vi "Alicat Simplified Driver Example_Multiple Devices with Setpoint.vi"() -> ()   [LabVIEW 2015]
doc: "Simplified example program for initializing the COM port, determining the data frame of up to 26 Alicats, acquiring the data of the same number of Alicats, displaying the data of the one with the selected unit ID, and writing a setpoint to the same selected unit ID.\n\nThis is a slightly more feature rich version of the Alicat Simplified Driver Example, and contains an example of a method for interfacing with up to 26 Alicats on a single COM port by means of for loops with shift registers to handle sequential commands to each included Alicat. This also contains a method to write a setpoint to the same selected unit.\n\nIf coding for multiple Alicats on a single COM port without the use of for loops with shift registers, ensure that each Alicat command is executed sequentially. Alicat's RS-232/485 does not work if multiple devices are responding simultaneously."
panel:
  in  "Setpoint (for \ndevice selected)":dbl format="%_4g"
  out "Meas. Data (for active device)":T1
  in  "Active Device":u16(ring) items=["A", "B", "C"]
  in  "Device ID's \nto Include:":T2={"A"=TRUE, "B"=FALSE, "C"=FALSE, "D"=FALSE, "E"=FALSE, "F"=FALSE, "G"=FALSE, "H"=FALSE, "I"=FALSE, "J"=FALSE, "K"=FALSE, "L"=FALSE, "M"=FALSE, "N"=FALSE, "O"=FALSE, "P"=FALSE, "Q"=FALSE, "R"=FALSE, "S"=FALSE, "T"=FALSE, "U"=FALSE, "V"=FALSE, "W"=FALSE, "X"=FALSE, "Y"=FALSE, "Z"=FALSE}
  in  "Minimum time between \nreadings [ms] (all units)":u32
  out "Elapsed Time [ms]\n(all units)":dbl caption="Elapsed Time (s)"
  in  "End Program":bool
  out "Error Text":string
  out "Error Present":bool
  out "Range Exceeded":bool
  in  "COM Port Settings":T3={"Baud Rate"=enum."19200", "VISA Sesssion In"="COM1"}
  # "Totalizer Timer"
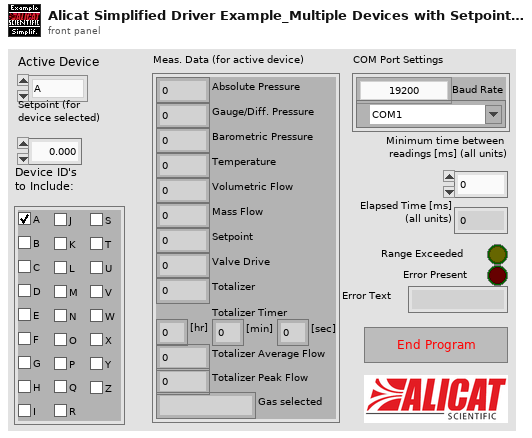
[diagram p1: front panel]
types:
  T1 = cluster{"Absolute Pressure":dbl, "Gauge/Diff. Pressure":dbl, "Barometric Pressure":dbl, "Temperature":dbl, "Volumetric Flow":dbl, "Mass Flow":dbl, "Setpoint":dbl, "Valve Drive":dbl, "Totalizer":dbl, "[hr]":dbl, "[min]":dbl, "[sec]":dbl, "Totalizer Average Flow":dbl, "Totalizer Peak Flow":dbl, "Gas selected":string}
  T2 = cluster{"A":bool, "B":bool, "C":bool, "D":bool, "E":bool, "F":bool, "G":bool, "H":bool, "I":bool, "J":bool, "K":bool, "L":bool, "M":bool, "N":bool, "O":bool, "P":bool, "Q":bool, "R":bool, "S":bool, "T":bool, "U":bool, "V":bool, "W":bool, "X":bool, "Y":bool, "Z":bool}
  T3 = cluster{"Baud Rate":enum8{"2400", "9600", "19200", "38400", "57600", "115200", "Unknown"}, "VISA Sesssion In":refnum<visa-resource-name>}
  T4 = cluster{"Unit ID":string, "Baud Rate":enum8{"2400", "9600", "19200", "38400", "57600", "115200", "Unknown"}, "VISA Sesssion In":refnum<visa-resource-name>}
  T5 = enum8{"2400", "9600", "19200", "38400", "57600", "115200", "Unknown"}
  T6 = cluster{"Absolute Pressure":bool, "Gauge/Diff. Pressure":bool, "Barometric Pressure":bool, "Temperature":bool, "Volumetric":bool, "Mass":bool, "Setpoint":bool, "Valve Drive":bool, "Totalizer":bool, "Totalizer Timer":bool, "Totalizer Average Flow":bool, "Totalizer Peak Flow":bool, "Gas Selected":bool, "Tot. Timer Format":u16}
  T7 = cluster{"Controller Full Scale":dbl, "Controller Select":u16, "Control Range":enum16{"Normal", "Inverted", "Bidirectional", "Unknown"}}
  T8 = cluster{"Controller Full Scale":dbl, "Controller Select":u16, "Control Range":enum16{"Normal", "Inverted", "Bidirectional", "Unknown"}}[]
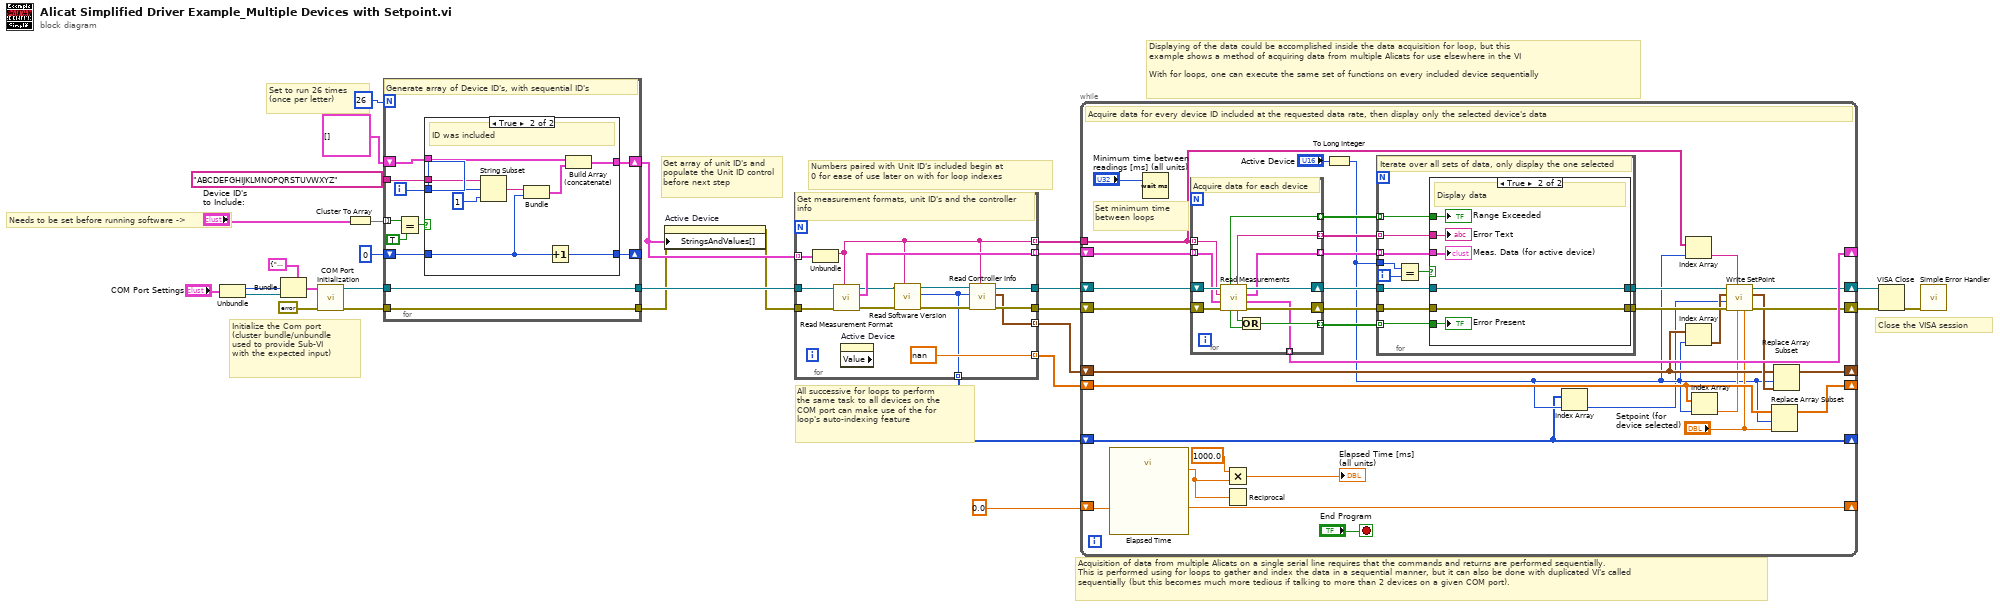
[diagram p0: block diagram]
diagram:
  # "All successive for loops to perform\nthe same task to all devices on the\nCOM port can make use of the for\nloop's auto-indexing feature"
  # "Set to run 26 times\n(once per letter)"
  # "Acquisition of data from multiple Alicats on a single serial line requires that the commands and returns are performed sequentially.\nThis is performed using for loops to gather and index the data in a sequential manner, but it can also be done with duplicated VI's called\nsequentially (but this becomes much more tedious if talking to more than 2 devices on a given COM port)."
  # "Numbers paired with Unit ID's included begin at\n0 for ease of use later on with for loop indexes"
  # "Displaying of the data could be accomplished inside the data acquisition for loop, but this\nexample shows a method of acquiring data from multiple Alicats for use elsewhere in the VI\n\nWith for loops, one can execute the same set of functions on every included device sequentially"
  # "Get array of unit ID's and populate the Unit ID control before next step"
  # "Needs to be set before running software ->"
  # "Close the VISA session"
  # "Initialize the Com port\n(cluster bundle/unbundle\nused to provide Sub-VI \nwith the expected input)"
  n1 = Unbundle("COM Port Settings") -> ("Baud Rate"=w22:T5, "VISA Sesssion In"=w21:refnum<visa-resource-name>)
  n2 = Bundle(cluster=T4 {"Unit ID"="A", "Baud Rate"=enum."19200", "VISA Sesssion In"="COM1"} ("Communication Settings"), "Baud Rate"=w22, "VISA Sesssion In"=w21) -> (w20:T4)  [unwired: 1 in]
  n3 = call "COM Port Initialization.vi"("error in (no error)"=errorcluster {"status"=FALSE, "code"=0, "source"=""}, "Communication Settings"=w20) -> ("error out"=w13:errorcluster, "VISA Session Out"=w12:refnum<visa-resource-name>)  [unwired: 8 in]
  n4 = Cluster To Array(cluster="Device ID's \nto Include:") -> (array=w16:bool[])
  n5 = for {
    N: 26 -> [_]
    tunnel: "ABCDEFGHIJKLMNOPQRSTUVWXYZ" -> [w40]
    tunnel: w16 -> [w33] mode=indexing
    shift-right: [w32] -> _
    shift-left: u16 0 ("length (rest)") -> [w38]
    shift-right: [w37] -> w10
    shift-left: cluster{string, u16}[] [] -> [w36]
    tunnel: w13 -> [w31]
    tunnel: w12 -> [w30]
    tunnel: [w31] -> w3
    tunnel: [w30] -> w11
    i -> [w39]
    # "Generate array of Device ID's, with sequential ID's"
    n6 = Equal?(x=w33, y=TRUE) -> (x = y?=w35:bool)
    n7 = case shown="True" w35 {
      tunnel: w40 -> [_ w51]
      tunnel: w39 -> [_ w50]
      tunnel: w38 -> [w41 w43]
      tunnel: [w42 w46] -> w37
      tunnel: w36 -> [w42 w44]
      tunnel: [w41 w47] -> w32
      frame False {
        # "ID was not included"
      }
      frame True {
        # "ID was included"
        n8 = String Subset(string=w51, offset (0)=w50, length (rest)=1 ("length (rest)")) -> (substring=w48:string)
        n9 = Bundle(w48, "length (rest)"=w43) -> (w45:cluster{string, "length (rest)":u16})  [unwired: 1 in]
        n10 = Increment(x=w43) -> (x+1=w47:u16)
        n11 = Build Array (concatenate)(w44, w45) -> (w46:cluster{string, "length (rest)":u16}[])
      }
    }
  }
  n12 = property on="Active Device" class="Ring (strict)"(error in=w3, "StringsAndValues[]"=w10) -> (error out=w2:errorcluster)  [unwired: 1 in, 1 out]
  n13 = for {
    tunnel: w11 -> [w64]
    tunnel: [w61] -> w7
    tunnel: w2 -> [w65]
    tunnel: [w60] -> w6
    tunnel: w10 -> [w62] mode=indexing
    tunnel: [w63] -> w9 mode=indexing
    tunnel: [w53] -> w8 mode=indexing
    tunnel: [w59] -> w5 mode=indexing
    tunnel: [nan ("Setpoint")] -> w4 mode=indexing
    tunnel: [w52] -> w1 mode=indexing
    # "Get measurement formats, unit ID's and the controller info"
    n14 = Unbundle(w62) -> (w53:string)  [unwired: 1 out]
    n15 = call "Read Measurement Format.vi"("Unit ID (A)"=w53, "error in"=w65, "VISA Session In"=w64) -> ("error out"=w56:errorcluster, "Data Frame Format"=w63:T6, "VISA Session Out"=w57:refnum<visa-resource-name>)  [unwired: 6 in]
    n16 = property on="Active Device" class="Ring (strict)" props=["Value"]() -> ()  [unwired: 2 in, 3 out]
    n17 = call "Read Software Version.vi"("Unit ID (A)"=w53, "error in"=w56, "VISA Session In"=w57) -> ("error out"=w55:errorcluster, "Software Version"=w52:u8, "VISA Session Out"=w54:refnum<visa-resource-name>)  [unwired: 6 in]
    n18 = call "Read Controller Info.vi"("Unit ID (A)"=w53, "error in"=w55, "Software Version"=w52, "VISA Session In"=w54) -> ("error out"=w60:errorcluster, "Controller Info out"=w59:T7, "VISA Session Out"=w61:refnum<visa-resource-name>)  [unwired: 4 in, 1 out]
  }
  n19 = while {
    shift-right: [w97] -> _
    shift-left: 0.0 ("Set Start Time (s)") -> [w100]
    shift-right: [w79] -> w25
    shift-left: w6 -> [w99]
    shift-right: [w80] -> w26
    shift-left: w7 -> [w98]
    tunnel: w8 -> [w71]
    shift-right: [w83] -> _
    shift-left: w9 -> [w91]
    shift-right: [w78] -> _
    shift-left: w5 -> [w76]
    shift-right: [w74] -> _
    shift-left: w4 -> [w73]
    shift-right: [w66] -> _
    shift-left: w1 -> [w66]
    stop <- "End Program" stop-if-true
    # "Set minimum time\nbetween loops"
    # "Acquire data for every device ID included at the requested data rate, then display only the selected device's data"
    n20 = call "Elapsed Time"("Set Start Time (s)"=w100) -> ("Get Start Time (s)"=w97:dbl, "Elapsed Time (s)"=w93:dbl)  [unwired: 11 in, 6 out]
    n21 = Wait (ms)(milliseconds to wait="Minimum time between \nreadings [ms] (all units)") -> ()  [unwired: 1 out]
    n22 = for {
      shift-right: [w129] -> w90
      shift-left: w99 -> [w132]
      shift-right: [w130] -> w89
      shift-left: w98 -> [w131]
      tunnel: w91 -> [w126] mode=indexing
      tunnel: w71 -> [w125] mode=indexing
      tunnel: [w124] -> w88 mode=indexing
      tunnel: [w123] -> w86 mode=indexing
      tunnel: [w122] -> w85 mode=indexing
      tunnel: [w121] -> w84 mode=indexing
      tunnel: [w120] -> w83 mode=indexing
      # "Acquire data for each device"
      n23 = call "Read Measurements.vi"("error in"=w132, "Data Frame Format In"=w126, "Unit ID (A)"=w125, "VISA Session In"=w131) -> ("error out"=w129:errorcluster, "Data Frame Format Out"=w120:T6, "Data Cluster"=w123:T1, "VISA Session Out"=w130:refnum<visa-resource-name>, "Unknown Dataframe Info"=w128:bool, "Error/Overrange/Unknown String"=w122:string, "Error Present"=w127:bool, "Range Exceeded"=w121:bool)
      n24 = Or(x=w128, y=w127) -> (x .or. y?=w124:bool)
    }
    n25 = Multiply(x=1000.0 ("y"), y=w93) -> (x*y=→"Elapsed Time [ms]\n(all units)":dbl)
    n26 = Reciprocal(x=w93) -> ()  [unwired: 1 out]
    n27 = To Long Integer(number="Active Device") -> (32bit integer=w68:i32)
    n28 = for {
      tunnel: w90 -> [w103]
      tunnel: [w102] -> w81
      tunnel: w89 -> [w104]
      tunnel: [w101] -> w82
      tunnel: w88 -> [w109] mode=indexing
      tunnel: w68 -> [w111]
      tunnel: w86 -> [w108] mode=indexing
      tunnel: w85 -> [w107] mode=indexing
      tunnel: w84 -> [w106] mode=indexing
      i -> [w110]
      # "Iterate over all sets of data, only display the one selected"
      n29 = Equal?(x=w111, y=w110) -> (x = y?=w105:bool)
      n30 = case shown="True" w105 {
        tunnel: w109 -> [_ w119]
        tunnel: w108 -> [_ w114]
        tunnel: w107 -> [_ w118]
        tunnel: w106 -> [_ w117]
        tunnel: w104 -> [w113 w115]
        tunnel: w103 -> [w112 w116]
        tunnel: [w112 w116] -> w102
        tunnel: [w113 w115] -> w101
        frame False {
          # "Do nothing"
        }
        frame True {
          # "Display data"
          "Range Exceeded" <- w117
          "Error Present" <- w119
          "Error Text" <- w118
          "Meas. Data (for active device)" <- w114
        }
      }
    }
    n31 = Index Array(array=w66, index=w68) -> (element=w67:u8)
    n32 = Index Array(array=w71, index=w68) -> (element=w70:string)
    n33 = Index Array(array=w76, index=w68) -> (element=w75:T7)
    n34 = Index Array(array=w73, index=w68) -> (element=w72:dbl)
    n35 = call "Write SetPoint.vi"("Setpoint"="Setpoint (for \ndevice selected)", "Previous Setpoint"=w72, "Unit ID (A)"=w70, "error in"=w81, "Software Version"=w67, "Controller Info out"=w75, "VISA Session In"=w82) -> ("error out"=w79:errorcluster, "Controller Info out"=w77:T7, "VISA Session Out"=w80:refnum<visa-resource-name>)  [unwired: 1 in, 1 out]
    n36 = Replace Array Subset(array=w73, new element="Setpoint (for \ndevice selected)", index=w68) -> (w74:dbl[])
    n37 = Replace Array Subset(array=w76, new element=w77, index=w68) -> (w78:T8)
  }
  n38 = VISA Close(VISA resource name=w26, error in (no error)=w25) -> (error out=w27:errorcluster)
  n39 = call <vilib>:"Simple Error Handler.vi"("error in (no error)"=w27) -> ()  [unwired: 4 in, 5 out]
